vi "ExtractName_ofSWFfile_fromHTML_href.vi"(7 "offset in":i32, 8 "error in (no error)":errorcluster, 10 "Identifying_String":string="href=", 11 "Dencrypted HTML":string) -> (0 "error out":errorcluster, 1 "AllText":string, 2 "Found?":bool, 3 "fileName":string, 4 "FolderName":string, 5 "offset past match":i32)   [LabVIEW 2016]
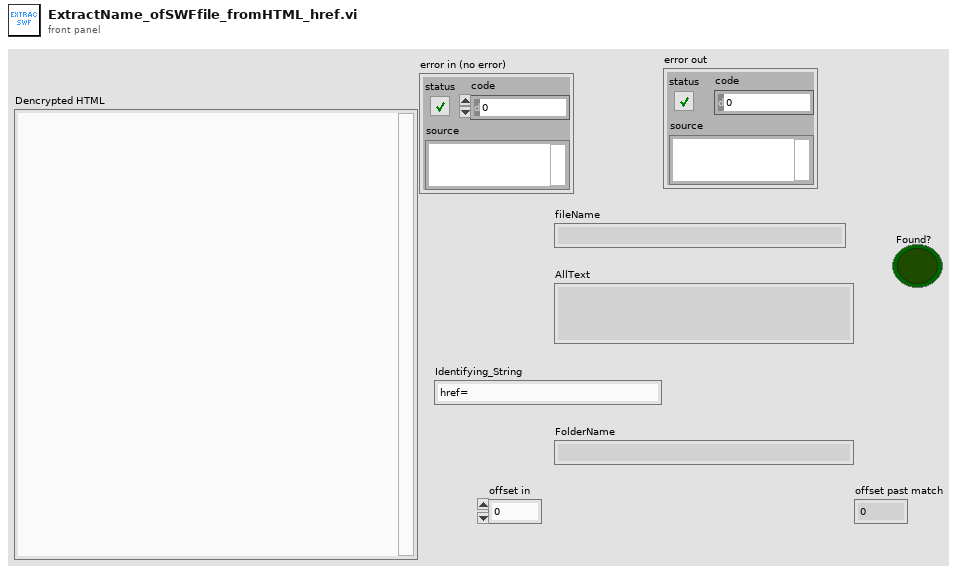
[diagram p1: front panel]
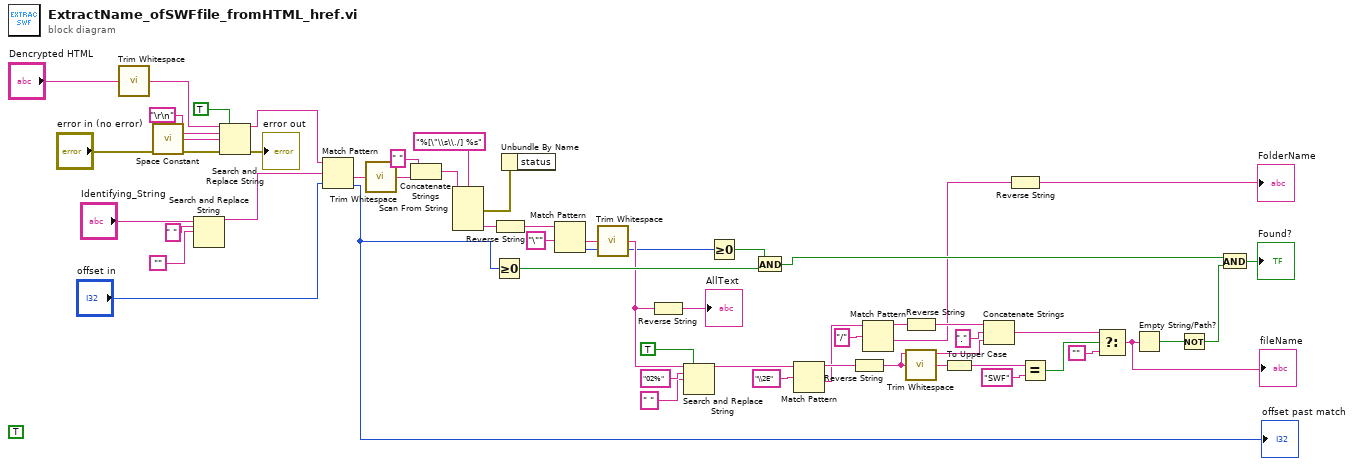
[diagram p0: block diagram]
diagram:
  (unwired) TRUE ("replace all? (F)")
  n1 = call <vilib>:"Trim Whitespace.vi"("string"="Dencrypted HTML") -> ("trimmed string"=w51:string)  [unwired: 1 in]
  n2 = call <vilib>:"Space Constant.vi"() -> ("String"=w43:string)
  n3 = Search and Replace String(input string="Identifying_String", search string=" ", replace string="") -> (result string=w4:string)  [unwired: 5 in, 3 out]
  n4 = Search and Replace String(replace all?=TRUE ("replace all? (F)"), input string=w51, search string="\r\n", replace string=w43, error in="error in (no error)") -> (result string=w53:string, error out=→"error out":errorcluster)  [unwired: 3 in, 2 out]
  n5 = Match Pattern(string=w53, regular expression=w4, offset (0)="offset in") -> (after substring=w38:string, offset past match=w46:i32)  [unwired: 2 out]
  "offset past match" <- w46
  n6 = call <vilib>:"Trim Whitespace.vi"("string"=w38) -> ("trimmed string"=w2:string)  [unwired: 1 in]
  n7 = Concatenate Strings(" " ("search string"), w2) -> (w1:string)
  n8 = Scan From String(format string="%[\"\\s\\./] %s", input string=w1) -> (error out=w16:errorcluster, output 2=w21:string)  [unwired: 5 in, 2 out]
  n9 = Greater Or Equal To 0?(x=w46) -> (x >= 0?=w45:bool)
  n10 = Reverse String(1:w21) -> (0:w13:string)
  n11 = Unbundle By Name(w16) -> ()  [unwired: 1 out]
  n12 = Match Pattern(string=w13, regular expression="\"") -> (after substring=w14:string, offset past match=w11:i32)  [unwired: 1 in, 2 out]
  n13 = call <vilib>:"Trim Whitespace.vi"("string"=w14) -> ("trimmed string"=w12:string)  [unwired: 1 in]
  n14 = Reverse String(1:w12) -> (0:→"AllText":string)
  n15 = Search and Replace String(replace all?=TRUE ("replace all? (F)"), input string=w12, search string="02%", replace string=" " ("replace string (\"\")")) -> (result string=w17:string)  [unwired: 4 in, 3 out]
  n16 = Greater Or Equal To 0?(x=w11) -> (x >= 0?=w10:bool)
  n17 = And(x=w10, y=w45) -> (x .and. y?=w40:bool)
  n18 = Match Pattern(string=w17, regular expression="\\2E") -> (before substring=w30:string, after substring=w29:string)  [unwired: 1 in, 2 out]
  n19 = Reverse String(1:w30) -> (0:w24:string)
  n20 = Match Pattern(string=w29, regular expression="/") -> (before substring=w27:string, after substring=w8:string)  [unwired: 1 in, 2 out]
  n21 = Reverse String(1:w27) -> (0:w26:string)
  n22 = call <vilib>:"Trim Whitespace.vi"("string"=w24) -> ("trimmed string"=w37:string)  [unwired: 1 in]
  n23 = To Upper Case(1:w37) -> (0:w36:string)
  n24 = Concatenate Strings(w26, "." ("string"), w24) -> (w22:string)
  n25 = Reverse String(1:w8) -> (0:→"FolderName":string)
  n26 = Equal?(x=w36, y="SWF") -> (x = y?=w34:bool)
  n27 = Select(t=w22, s=w34, f="") -> (s? t:f=w25:string)
  "fileName" <- w25
  n28 = Empty String/Path?(string/path=w25) -> (empty?=w42:bool)
  n29 = Not(x=w42) -> (.not. x?=w41:bool)
  n30 = And(x=w40, y=w41) -> (x .and. y?=→"Found?":bool)
